vi "弹窗-设置串口.vi"(10 "串口探头地址":u16[](array[numeric]), 11 "串口通信单元-改动项引用[]":refnum<vi>[](array[refnum])) -> ()   [LabVIEW 2017]
panel:
  in  "标志-配置改变?":bool=TRUE
  in  "应用于探头":bool
  in  "波特率":enum16{"9600", "19200"}(ring)
  in  "COM口":refnum<visa-resource-name>
  in  "应用于软件":bool
  in  "取消":bool
  out "信号-关闭窗口":bool=TRUE
  # "串口通信设置"
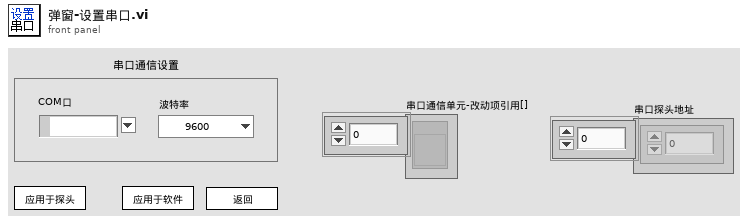
[diagram p1: front panel]
types:
  T1 = typedef "簇-输入.ctl" = cluster{"配置文件动作":T2, "数据输入":variant}
  T2 = typedef "枚举-配置文件动作.ctl" = enum16{"初始化加载配置", "读取配置", "写入-屏幕键盘", "写入-静音延迟", "写入-主要探头类型", "写入-串口配置", "写入-累积定时", "写入-导出定时", "保存配置到文件"}
  T3 = enum32{"Invalid", "Standard", "Closed", "Hidden", "Minimized", "Maximized"}
  T4 = typedef "串口模块输入.ctl" = cluster{"串口动作类型":T5, "串口配置":T6, "数据输入":variant}
  T5 = typedef "串口动作类型.ctl" = enum16{"读测量值", "设置报警值", "设置地址", "设置系数", "广播修改波特率", "关闭串口"}
  T6 = typedef "串口配置.ctl" = cluster{"COM口":refnum<visa-resource-name>, "波特率":enum16{"9600", "19200"}, "探头地址(U8)":u8}
  T7 = typedef "簇-配置文件内容.ctl" = cluster{"调试模式？":bool, "屏幕键盘？":bool, "软件版本":string, "静音延迟 s":u16, "主要探头类型":T8, "串口配置":cluster{"COM口":refnum<visa-resource-name>, "波特率":enum16{"9600", "19200"}, "读写超时ms":i16, "丢包判定次数":i16}, "定时配置-累积分段":T9, "定时配置-自动导出":cluster{"定时配置-自动导出":T9, "分别导出?":bool}}
  T8 = typedef "枚举-主要探头类型.ctl" = enum16{"网络探头", "串口探头"}
  T9 = typedef "簇-定时配置.ctl" = cluster{"定时模式":enum16{"绝对时间", "相对时间"}, "单位":enum16{"年", "月", "日", "时", "分"}, "间隔":u8, "目标时刻":timestamp}
  T10 = typedef "改动项选择.ctl" = enum16{"未改动", "改动-启用状态", "改动-探头信息", "改动-报警限值", "动作-手动静音", "动作-重启累积时段", "动作-累积删除", "动作-重连"}
  T11 = typedef "改动项.ctl" = cluster{"改动项选择":T10, "启用？":bool, "探测器信息":T12}
  T12 = typedef "探测器信息.ctl" = cluster{"网络地址":string, "名称":string, "备注":string, "累积剂量":dbl, "累积限值":dbl, "硬件剂量率限值":T13, "剂量率限值1":dbl, "剂量率限值2":dbl, "报警方式":T14}
  T13 = typedef "探头剂量率限值选择.ctl" = enum16{"一级限值", "二级限值"}
  T14 = typedef "报警方式选择.ctl" = enum16{"常报警", "自动静音", "手动静音"}
  T15 = cluster{"COM口":refnum<visa-resource-name>, "波特率":enum16{"9600", "19200"}, "读写超时ms":i16, "丢包判定次数":i16}
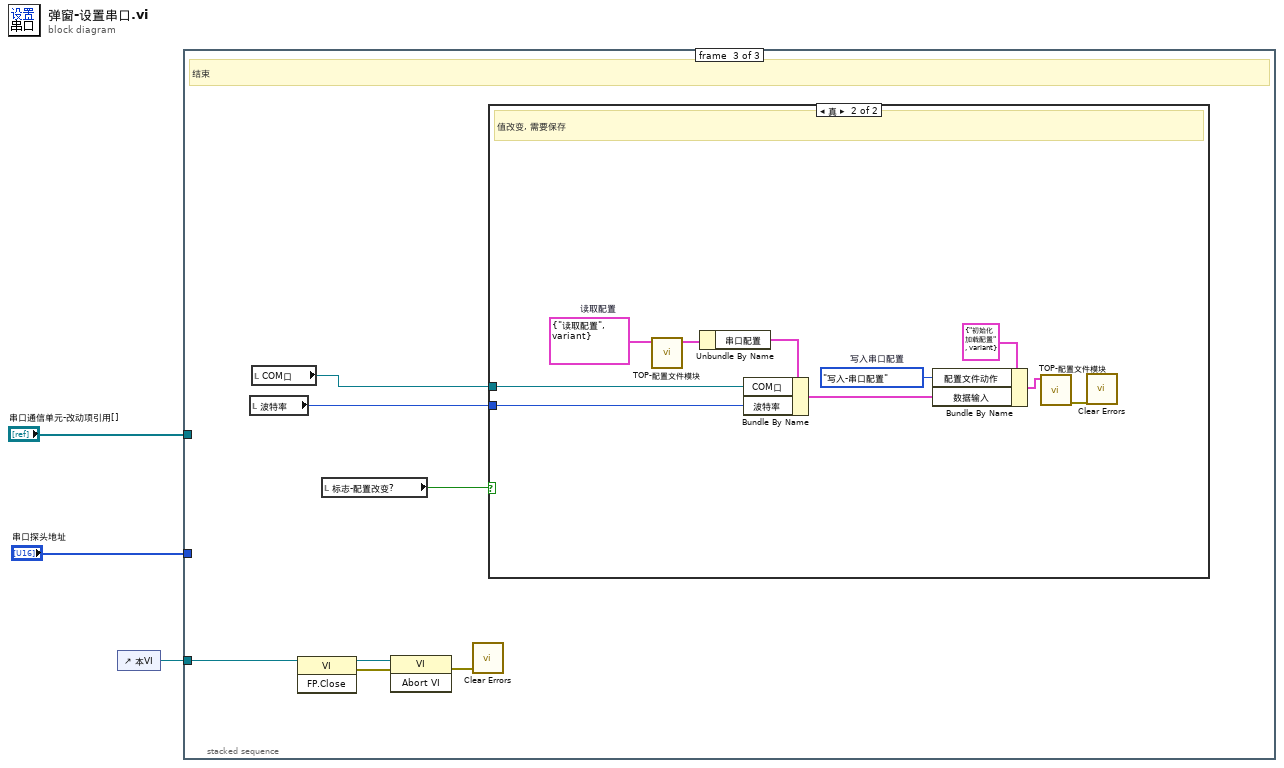
[diagram p0: block diagram]
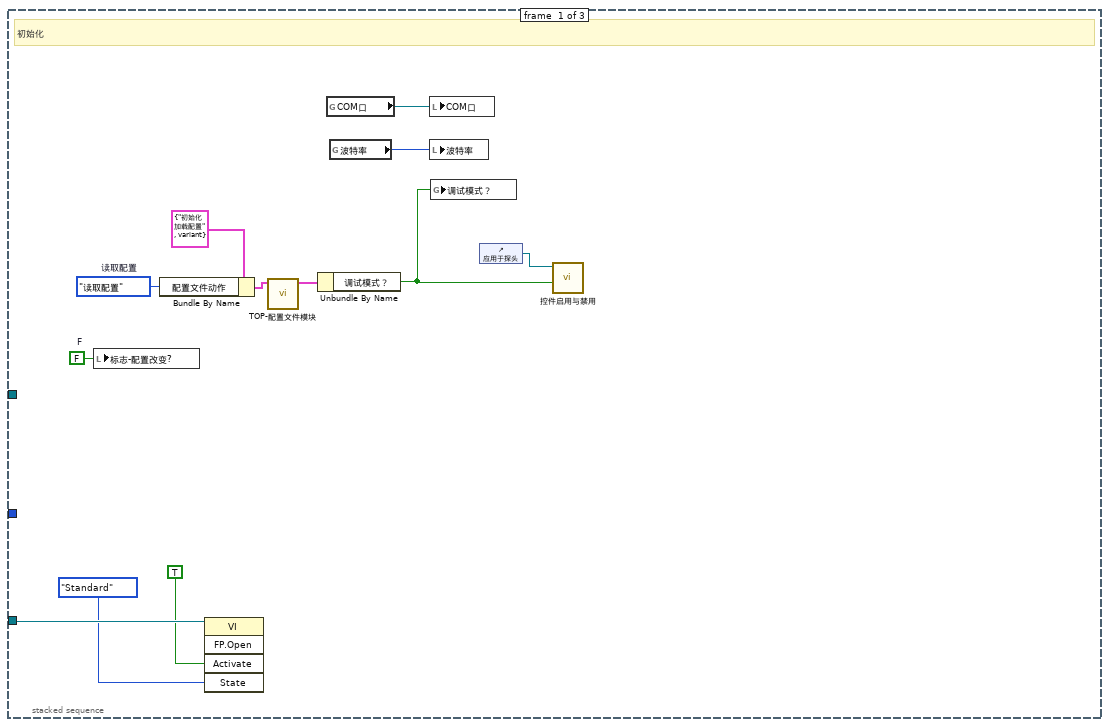
[diagram p2: hidden frame]
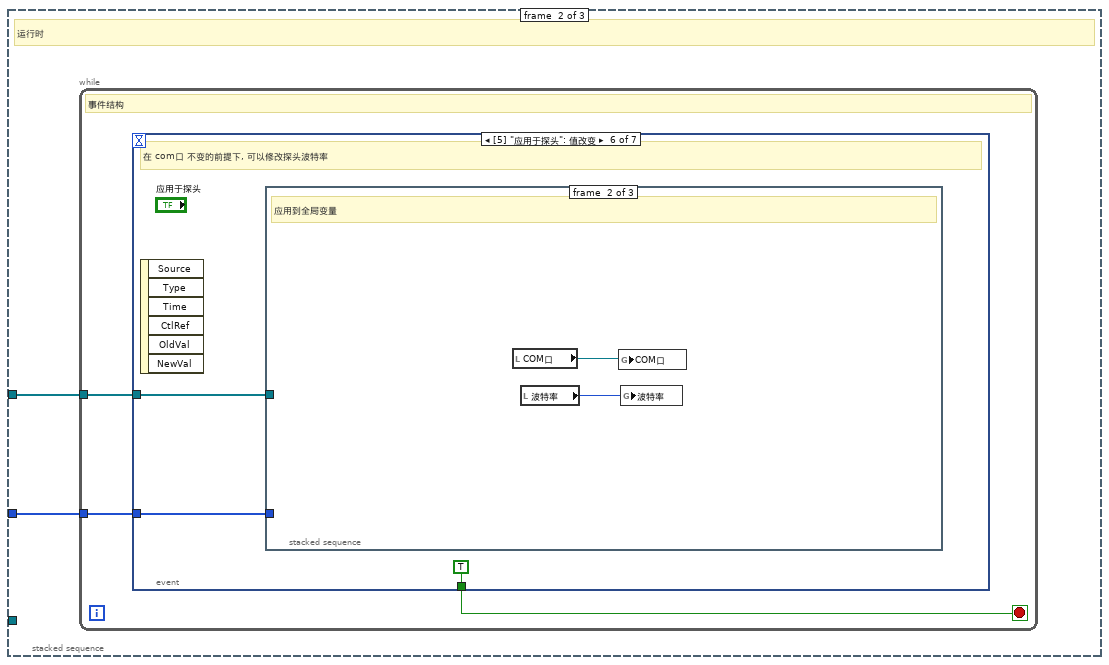
[diagram p3: hidden frame]
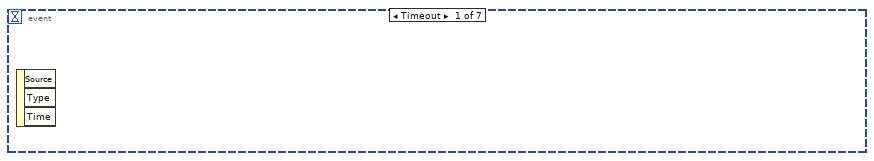
[diagram p4: hidden frame]
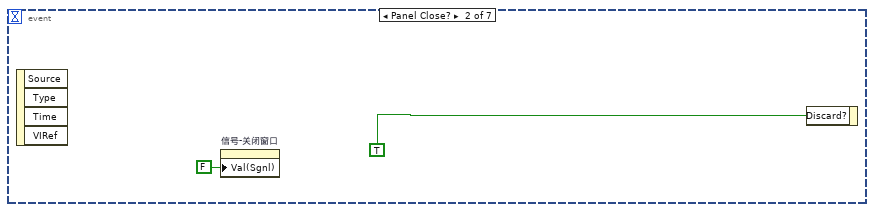
[diagram p5: hidden frame]
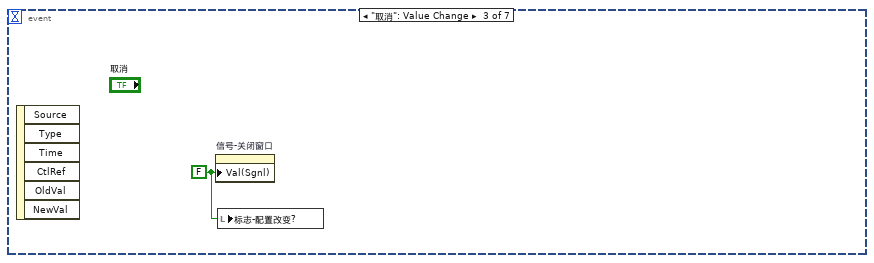
[diagram p6: hidden frame]
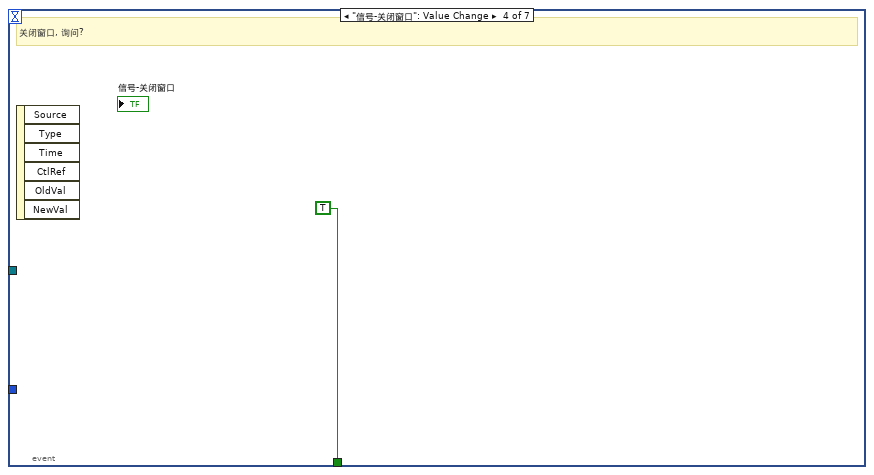
[diagram p7: hidden frame]
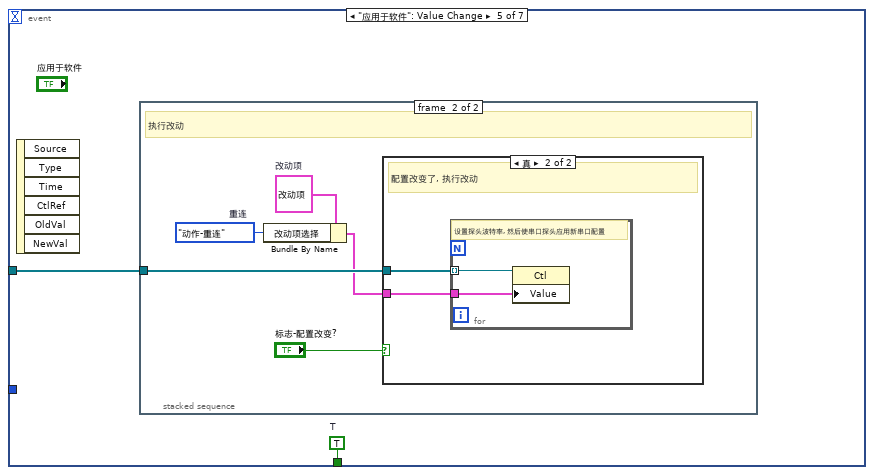
[diagram p8: hidden frame]
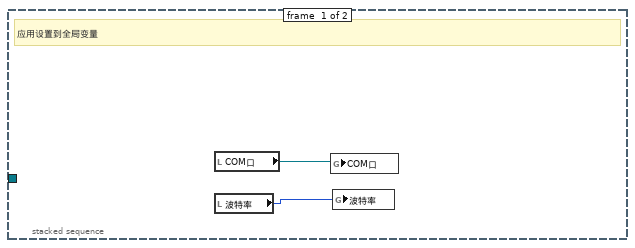
[diagram p9: hidden frame]
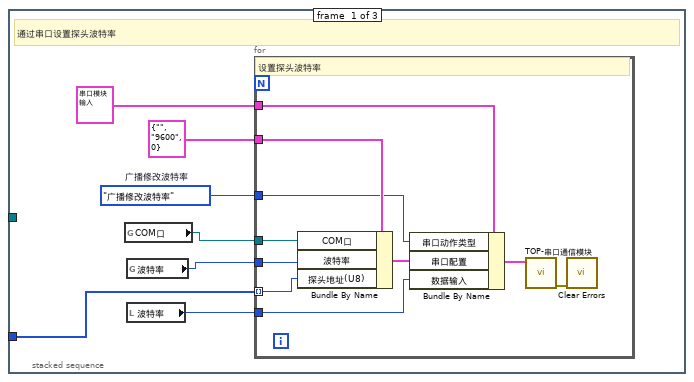
[diagram p11: hidden frame]
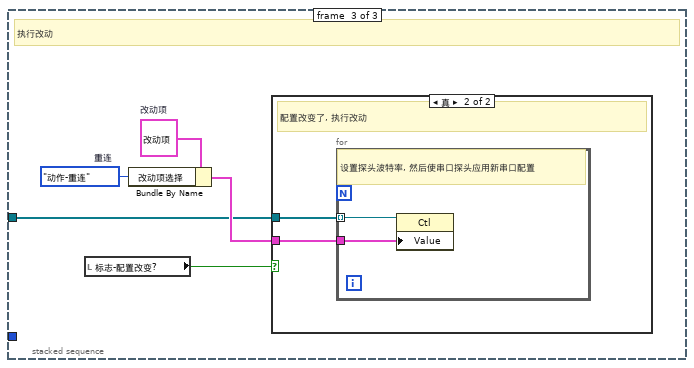
[diagram p12: hidden frame]
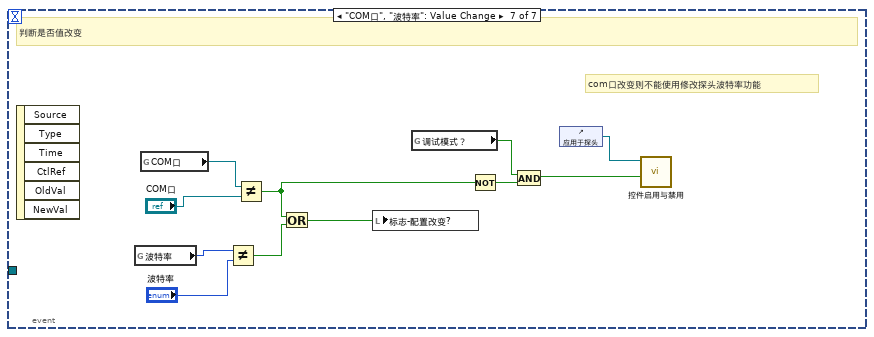
[diagram p14: hidden frame]
diagram:
  n1 = control-ref of="本VI"() -> (w3:refnum<vi>)
  n2 = stacked-sequence {
    tunnel: w3 -> [w15 _ w86]
    tunnel: "串口通信单元-改动项引用[]" -> [_ w17 _]
    tunnel: "串口探头地址" -> [_ w16 _]
    frame #0 {
      w5 = FALSE  # F
      w9 = 枚举-配置文件动作."读取配置"  # 读取配置
      # "初始化"
      n3 = local write "标志-配置改变?"(w5) -> ()
      n4 = Bundle By Name(cluster=T1 {"配置文件动作"=enum."初始化加载配置", "数据输入"=variant} ("输入"), "配置文件动作"=w9) -> (w8:T1)
      n5 = invoke class="VI" method="FP.Open"(reference=w15, "Activate"=TRUE ("激活？"), "State"=T3."Standard" ("状态")) -> ()  [unwired: 2 in, 5 out]
      n6 = call "TOP-配置文件模块.vi"("输入"=w8) -> ("配置文件"=w10:T7)  [unwired: 9 in, 1 out]
      n7 = Unbundle By Name(w10) -> ("调试模式？"=w4:bool)
      n8 = global read "全局变量-35点监测.vi" "COM口"() -> (w12:refnum<visa-resource-name>)
      n9 = global read "全局变量-35点监测.vi" "波特率"() -> (w11:enum16{"9600", "19200"})
      n10 = local write "COM口"(w12) -> ()
      n11 = local write "波特率"(w11) -> ()
      n12 = global write "全局变量-35点监测.vi" "调试模式？"(w4) -> ()
      n13 = control-ref of="应用于探头"() -> (w6:refnum<vi>)
      n14 = call "控件启用与禁用.vi"("启用？"=w4, "控件引用"=w6) -> ()  [unwired: 9 in, 1 out]
    }
    frame #1 {
      # "运行时"
      n15 = while {
        tunnel: w17 -> [w19]
        tunnel: w16 -> [w18]
        stop <- w20 stop-if-true
        # "事件结构"
        n16 = event shown="[5] \"应用于探头\": 值改变" {
          selector: _ -> [_ _ _ _ _ _ _]
          dyn-events: _ -> [_ _ _ _ _ _ _]
          timeout: _ -> [_ _ _ _ _ _ _]
          tunnel: [_ _ _ TRUE w25 TRUE ("T") _] -> w20
          tunnel: w19 -> [_ _ _ _ w26 w40 _]
          tunnel: w18 -> [_ _ _ _ _ w39 _]
          event Timeout {
            n17 = event-data() -> ()  [unwired: 1 in, 3 out]
          }
          event Panel Close? {
            n18 = event-data() -> ()  [unwired: 1 in, 4 out]
            n19 = property on="信号-关闭窗口" class="Bool (严格)"("Val(Sgnl)"=FALSE ("值(信号)")) -> ()  [unwired: 2 in, 2 out]
            n20 = event-data("Discard?"=TRUE ("放弃？")) -> ()  [unwired: 1 in, 1 out]
          }
          event "取消": Value Change {
            w23 = FALSE ("值(信号)")
            n21 = event-data() -> ()  [unwired: 1 in, 6 out]
            n22 = property on="信号-关闭窗口" class="Bool (严格)"("Val(Sgnl)"=w23) -> ()  [unwired: 2 in, 2 out]
            n23 = local write "标志-配置改变?"(w23) -> ()
          }
          event "信号-关闭窗口": Value Change {
            # "关闭窗口, 询问?"
            n24 = event-data() -> ()  [unwired: 1 in, 6 out]
          }
          event "应用于软件": Value Change {
            w25 = TRUE  # T
            n25 = event-data() -> ()  [unwired: 1 in, 6 out]
            n26 = stacked-sequence {
              tunnel: w26 -> [_ w33]
              frame #0 {
                # "应用设置到全局变量"
                n27 = local read "COM口"() -> (w28:refnum<visa-resource-name>)
                n28 = local read "波特率"() -> (w27:enum16{"9600", "19200"})
                n29 = global write "全局变量-35点监测.vi" "COM口"(w28) -> ()
                n30 = global write "全局变量-35点监测.vi" "波特率"(w27) -> ()
              }
              frame #1 {
                w31 = 改动项选择."动作-重连"  # 重连
                w32 = T11 {"改动项选择"=enum."未改动", "启用？"=FALSE, "探测器信息"={"网络地址"="", "名称"="", "备注"="", "累积剂量"=0.0, "累积限值"=0.0, "硬件剂量率限值"=enum."一级限值", "剂量率限值1"=0.0, "剂量率限值2"=0.0, "报警方式"=enum."常报警"}}  # 改动项
                # "执行改动"
                n31 = Bundle By Name(cluster=w32, "改动项选择"=w31) -> (w30:T11)
                n32 = case shown="真" "标志-配置改变?" {
                  tunnel: w33 -> [_ w35]
                  tunnel: w30 -> [_ w34]
                  frame False {
                    # "配置没变, 不改动"
                  }
                  frame True {
                    # "配置改变了, 执行改动"
                    n33 = for {
                      tunnel: w35 -> [w37] mode=indexing
                      tunnel: w34 -> [w36]
                      # "设置探头波特率, 然后使串口探头应用新串口配置"
                      n34 = property class="Ctl"(reference=w37, "Value"=w36) -> ()  [unwired: 1 in, 2 out]
                    }
                  }
                }
              }
            }
          }
          event "应用于探头": Value Change {
            # "在 com口 不变的前提下, 可以修改探头波特率"
            n35 = event-data() -> ()  [unwired: 1 in, 6 out]
            n36 = stacked-sequence {
              tunnel: w40 -> [_ _ w61]
              tunnel: w39 -> [w47 _ _]
              frame #0 {
                w42 = 串口动作类型."广播修改波特率"  # 广播修改波特率
                # "通过串口设置探头波特率"
                n37 = global read "全局变量-35点监测.vi" "COM口"() -> (w46:refnum<visa-resource-name>)
                n38 = global read "全局变量-35点监测.vi" "波特率"() -> (w45:enum16{"9600", "19200"})
                n39 = local read "波特率"() -> (w41:enum16{"9600", "19200"})
                n40 = for {
                  tunnel: w47 -> [w55] mode=indexing
                  tunnel: w46 -> [w54]
                  tunnel: w45 -> [w53]
                  tunnel: T6 {"COM口"="", "波特率"=enum."9600", "探头地址(U8)"=0} ("串口配置") -> [w52]
                  tunnel: T4 {"串口动作类型"=enum."读测量值", "串口配置"={"COM口"="", "波特率"=enum."9600", "探头地址(U8)"=0}, "数据输入"=variant} ("串口模块输入") -> [w51]
                  tunnel: w42 -> [w50]
                  tunnel: w41 -> [w49]
                  # "设置探头波特率"
                  n41 = Bundle By Name(cluster=w52, "COM口"=w54, "波特率"=w53, "探头地址(U8)"=w55) -> (w57:T6)
                  n42 = Bundle By Name(cluster=w51, "串口动作类型"=w50, "串口配置"=w57, "数据输入"=w49) -> (w56:T4)
                  n43 = call "TOP-串口通信模块.vi"("串口模块输入"=w56) -> ("error out"=w48:errorcluster)  [unwired: 9 in, 1 out]
                  n44 = call <vilib>:"Clear Errors.vi"("error in (no error)"=w48) -> ()  [unwired: 5 in, 2 out]
                }
              }
              frame #1 {
                # "应用到全局变量"
                n45 = local read "COM口"() -> (w59:refnum<visa-resource-name>)
                n46 = local read "波特率"() -> (w58:enum16{"9600", "19200"})
                n47 = global write "全局变量-35点监测.vi" "COM口"(w59) -> ()
                n48 = global write "全局变量-35点监测.vi" "波特率"(w58) -> ()
              }
              frame #2 {
                w63 = 改动项选择."动作-重连"  # 重连
                w64 = T11 {"改动项选择"=enum."未改动", "启用？"=FALSE, "探测器信息"={"网络地址"="", "名称"="", "备注"="", "累积剂量"=0.0, "累积限值"=0.0, "硬件剂量率限值"=enum."一级限值", "剂量率限值1"=0.0, "剂量率限值2"=0.0, "报警方式"=enum."常报警"}}  # 改动项
                # "执行改动"
                n49 = local read "标志-配置改变?"() -> (w60:bool)
                n50 = Bundle By Name(cluster=w64, "改动项选择"=w63) -> (w62:T11)
                n51 = case shown="真" w60 {
                  tunnel: w61 -> [_ w66]
                  tunnel: w62 -> [_ w65]
                  frame False {
                    # "配置没变, 不改动"
                  }
                  frame True {
                    # "配置改变了, 执行改动"
                    n52 = for {
                      tunnel: w66 -> [w68] mode=indexing
                      tunnel: w65 -> [w67]
                      # "设置探头波特率, 然后使串口探头应用新串口配置"
                      n53 = property class="Ctl"(reference=w68, "Value"=w67) -> ()  [unwired: 1 in, 2 out]
                    }
                  }
                }
              }
            }
          }
          event "COM口", "波特率": Value Change {
            # "com口改变则不能使用修改探头波特率功能"
            # "判断是否值改变"
            n54 = event-data() -> ()  [unwired: 1 in, 6 out]
            n55 = global read "全局变量-35点监测.vi" "波特率"() -> (w79:enum16{"9600", "19200"})
            n56 = global read "全局变量-35点监测.vi" "COM口"() -> (w76:refnum<visa-resource-name>)
            n57 = Not Equal?(x=w79, y="波特率") -> (x != y?=w75:bool)
            n58 = Not Equal?(x=w76, y="COM口") -> (x != y?=w72:bool)
            n59 = Or(x=w72, y=w75) -> (x .or. y?=w74:bool)
            n60 = local write "标志-配置改变?"(w74) -> ()
            n61 = global read "全局变量-35点监测.vi" "调试模式？"() -> (w69:bool)
            n62 = Not(x=w72) -> (.not. x?=w71:bool)
            n63 = And(x=w69, y=w71) -> (x .and. y?=w70:bool)
            n64 = control-ref of="应用于探头"() -> (w73:refnum<vi>)
            n65 = call "控件启用与禁用.vi"("启用？"=w70, "控件引用"=w73) -> ()  [unwired: 9 in, 1 out]
          }
        }
      }
    }
    frame #2 {
      # "结束"
      n66 = local read "波特率"() -> (w80:enum16{"9600", "19200"})
      n67 = local read "COM口"() -> (w82:refnum<visa-resource-name>)
      n68 = invoke class="VI" method="FP.Close"(reference=w86) -> (reference out=w85:refnum<vi>, error out=w84:errorcluster)  [unwired: 2 in, 1 out]
      n69 = local read "标志-配置改变?"() -> (w81:bool)
      n70 = invoke class="VI" method="Abort VI"(reference=w85, error in=w84) -> (error out=w83:errorcluster)  [unwired: 1 in, 2 out]
      n71 = call <vilib>:"Clear Errors.vi"("error in (no error)"=w83) -> ()  [unwired: 5 in, 2 out]
      n72 = case shown="真" w81 {
        tunnel: w82 -> [_ w92]
        tunnel: w80 -> [_ w91]
        frame False {
          # "值未变"
        }
        frame True {
          w89 = T1 {"配置文件动作"=enum."读取配置", "数据输入"=variant}  # 读取配置
          w95 = 枚举-配置文件动作."写入-串口配置"  # 写入串口配置
          # "值改变, 需要保存"
          n73 = call "TOP-配置文件模块.vi"("输入"=w89) -> ("配置文件"=w88:T7)  [unwired: 9 in, 1 out]
          n74 = Unbundle By Name(w88) -> ("串口配置"=w87:T15)
          n75 = Bundle By Name(cluster=w87, "COM口"=w92, "波特率"=w91) -> (w94:T15)
          n76 = Bundle By Name(cluster=T1 {"配置文件动作"=enum."初始化加载配置", "数据输入"=variant} ("输入"), "配置文件动作"=w95, "数据输入"=w94) -> (w96:T1)
          n77 = call "TOP-配置文件模块.vi"("输入"=w96) -> ("error out"=w90:errorcluster)  [unwired: 9 in, 1 out]
          n78 = call <vilib>:"Clear Errors.vi"("error in (no error)"=w90) -> ()  [unwired: 5 in, 2 out]
        }
      }
    }
  }
